vi "Configure Baud Rate.vi"(0 "UART Driver in":refnum<class "UART Driver.lvclass">, 1 "Controller Number":u8, 5 "Baud Rate":u32, 11 "error in":errorcluster) -> (4 "UART Driver out":refnum<class "UART Driver.lvclass">, 6 "Receive Data":string, 15 "error out":errorcluster)   [LabVIEW 2012, in "UART_Host_Driver.lvlib" / "UART Driver.lvclass"]
doc: "Configure the Port/s Baud Rate.\n\nMust call UART Initialize.vi, prior to calling UART Configure Baud Rate.vi.\n\nNote: Port Number 255 means to transmit to all of the ports configured in the UART Initialize.vi."
uses:
  UART Driver.lvclass
  FPGA/UART/UART_Command.ctl
  UART Driver.lvclass/UART Driver.ctl
  Typedefs/FPGA VI Reference.ctl
  <vilib>/Utility/error.llb/Error Cluster From Error Code.vi
  <vilib>/rvi/errors/niLvFpgaAdjustHostInterfaceError.vi
  <vilib>/rvi/interface/nirviMethod/nirviMethod.xnode
  UART_Host_Driver.lvlib
  <vilib>/FPGAPlugInAG/Dynamic/niLvFpga_WriteFifo_Dynamic.vi
  <vilib>/rvi/errors/niLvFpgaMergeErrorWithErrorCode.vi
  FPGA/UART/UART_Firmware.lvlib
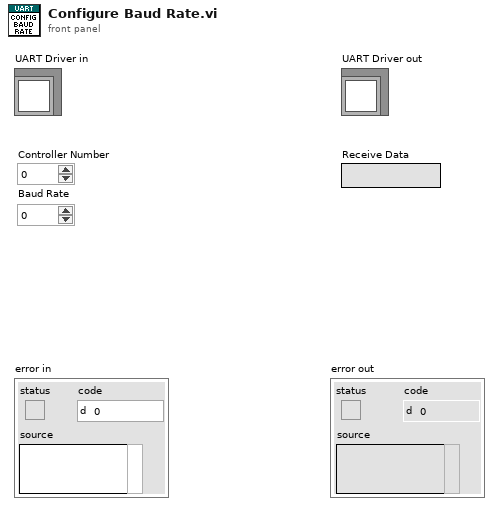
[diagram p1: front panel]
types:
  T1 = typedef "UART_Firmware.lvlib/UART_Command.ctl" = enum8{"None", "Tx", "SetBaud_High", "SetBaud_Low", "SetCharLength", "SetParity", "SetStopBits", "SetSpacing_High", "SetSpacing_Low"}
  T2 = typedef "UART_Host_Driver.lvlib/FPGA VI Reference.ctl" = refnum<k20>
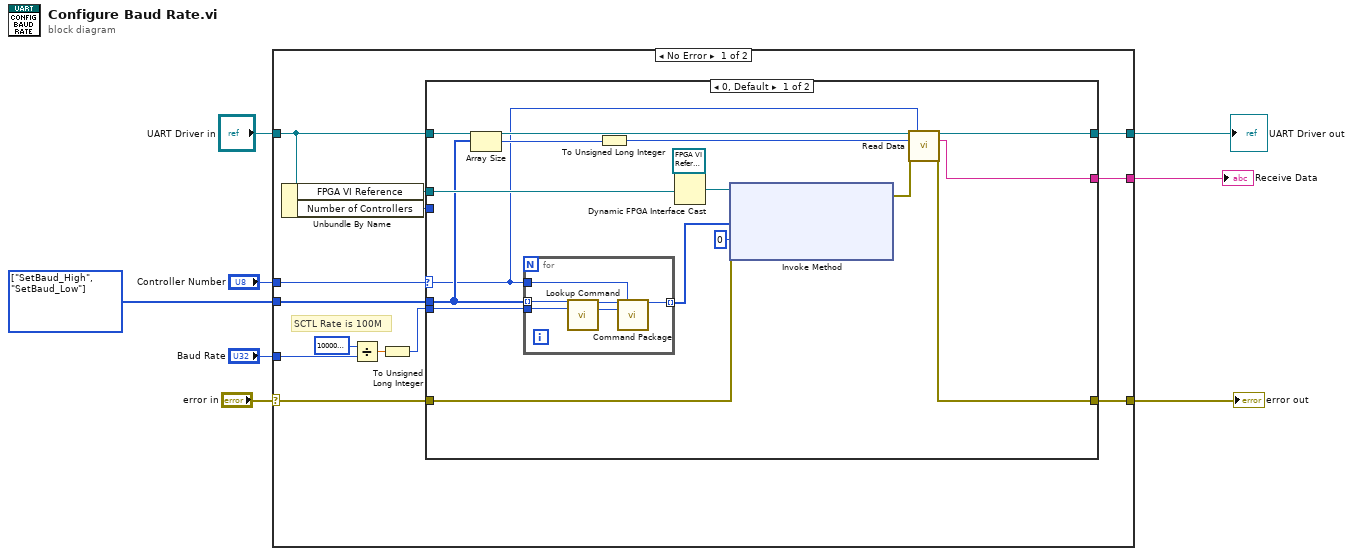
[diagram p0: block diagram]
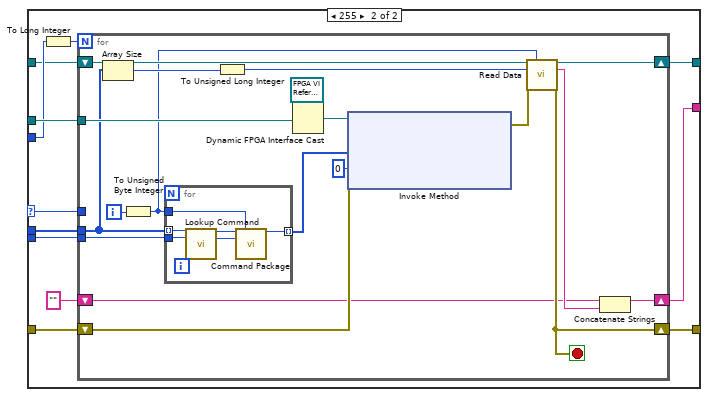
[diagram p2: hidden frame]
diagram:
  w1 = T1[] [enum."SetBaud_High", enum."SetBaud_Low"] items=["None", "Tx", "SetBaud_High", "SetBaud_Low", "SetCharLength", "SetParity", "SetStopBits", "SetSpacing_High", "SetSpacing_Low"] ("Input Parameters")
  n1 = case shown="No Error" "error in" {
    selector: "error in" -> [w20 w82]
    tunnel: [w17 w82] -> w7
    tunnel: [w18 w81] -> w5
    tunnel: "UART Driver in" -> [w19 w81]
    tunnel: "Baud Rate" -> [w12 _]
    tunnel: w1 -> [w15 _]
    tunnel: [w16 _] -> w3
    tunnel: "Controller Number" -> [w14 _]
    frame No Error {
      # "SCTL Rate is 100M"
      n2 = Unbundle By Name(w19) -> ("FPGA VI Reference"=w21:refnum<k20>, "Number of Controllers"=w13:u8)
      n3 = Divide(x=u32 100000000, y=w12) -> (x/y=w10:dbl)
      n4 = To Unsigned Long Integer(number=w10) -> (unsigned 32bit integer=w9:u32)
      n5 = case shown="0, Default" w14 {
        selector: w14 -> [w22 w49]
        tunnel: w9 -> [w37 w55]
        tunnel: w21 -> [w34 w54]
        tunnel: w20 -> [w31 w53]
        tunnel: w19 -> [w30 w46]
        tunnel: [w29 w52] -> w18
        tunnel: [w27 w51] -> w17
        tunnel: [w26 w44] -> w16
        tunnel: w15 -> [w25 w50]
        tunnel: w13 -> [_ w48]
        frame 0, Default {
          n6 = Array Size(array=w25) -> (size(s)=w24:i32)
          n7 = for {
            tunnel: w37 -> [w43]
            tunnel: [w40] -> w35 mode=indexing
            tunnel: w25 -> [w39] mode=indexing
            tunnel: w22 -> [w38]
            n8 = call "Lookup Command.vi"("UART_Command in"=w39, "Baud"=w43) -> ("UART_Command out"=w42:T1, "Numeric"=w41:u16)  [unwired: 12 in]
            n9 = call "Command Package.vi"("UART_Command"=w42, "Channel Number"=w38, "Cmd_data"=w41) -> ("Cmd_package"=w40:u32)  [unwired: 12 in]
          }
          n10 = To Unsigned Long Integer(number=w24) -> (unsigned 32bit integer=w23:u32)
          n11 = Dynamic FPGA Interface Cast(Session In=T2 refnum ("FPGA VI Reference"), Type=w34) -> (Session Out=w33:T2)
          n12 = xnode "Invoke Method"("FPGA VI Reference In"=w33, "error in"=w31, "Data"=w35, "Timeout (ms)"=0) -> ("error out"=w28:errorcluster)  [unwired: 2 out]
          n13 = call-dynamic "Read Data.vi"("UART Driver in"=w30, "Port Number"=w22, "Rx byte count"=w23, "error in"=w28) -> ("UART Driver out"=w29:refnum<class "UART Driver.lvclass">, "Receive Data"=w26:string, "error out"=w27:errorcluster)  [unwired: 9 in]
        }
        frame 255 {
          n14 = To Long Integer(number=w48) -> (32bit integer=w47:i32)
          n15 = for {
            N: w47 -> [_]
            tunnel: w55 -> [w74]
            tunnel: w54 -> [w71]
            tunnel: w50 -> [w65]
            tunnel: w49 -> [_]
            shift-right: [w67] -> w52
            shift-left: w46 -> [w62]
            shift-right: [w61] -> w51
            shift-left: w53 -> [w68]
            shift-right: [w58] -> w44
            shift-left: "" -> [w59]
            i -> [w57]
            stop <- w61 stop-if-true
            n16 = Array Size(array=w65) -> (size(s)=w64:i32)
            n17 = To Unsigned Byte Integer(number=w57) -> (unsigned 8bit integer=w56:u8)
            n18 = for {
              tunnel: w74 -> [w80]
              tunnel: [w77] -> w72 mode=indexing
              tunnel: w65 -> [w76] mode=indexing
              tunnel: w56 -> [w75]
              n19 = call "Lookup Command.vi"("UART_Command in"=w76, "Baud"=w80) -> ("UART_Command out"=w79:T1, "Numeric"=w78:u16)  [unwired: 12 in]
              n20 = call "Command Package.vi"("UART_Command"=w79, "Channel Number"=w75, "Cmd_data"=w78) -> ("Cmd_package"=w77:u32)  [unwired: 12 in]
            }
            n21 = To Unsigned Long Integer(number=w64) -> (unsigned 32bit integer=w63:u32)
            n22 = Dynamic FPGA Interface Cast(Session In=T2 refnum ("FPGA VI Reference"), Type=w71) -> (Session Out=w70:T2)
            n23 = xnode "Invoke Method"("FPGA VI Reference In"=w70, "error in"=w68, "Data"=w72, "Timeout (ms)"=0) -> ("error out"=w66:errorcluster)  [unwired: 2 out]
            n24 = call-dynamic "Read Data.vi"("UART Driver in"=w62, "Port Number"=w56, "Rx byte count"=w63, "error in"=w66) -> ("UART Driver out"=w67:refnum<class "UART Driver.lvclass">, "Receive Data"=w60:string, "error out"=w61:errorcluster)  [unwired: 9 in]
            n25 = Concatenate Strings(w59, w60) -> (w58:string)
          }
        }
      }
    }
    frame Error {
    }
  }
  "error out" <- w7
  "UART Driver out" <- w5
  "Receive Data" <- w3
